vi "XML Script - MathScript Call By Reference Node.vi"(1 "prefix (name)":string, 3 "in":i32=-1, 5 "name":string, 7 "mFilePath":path, 9 "linkIdentity":string, 11 "x":i32=-1, 12 "y":i32=-1, 14 "out":i32=-1) -> (4 "XML Script Command - SubVI":string, 10 "name (wire source)":string)   [LabVIEW 2020]
doc: "linkIdentity: <MFileName>:<FunctionName>\nExample: foo.m:foo"
uses:
  <vilib>/_script/XML Scripting/XML Script Attribute.ctl
  <vilib>/_script/XML Scripting/XML Script Tag.ctl
  <vilib>/_script/XML Scripting/XML Script - PathToXMLString.vi
panel:
  # "position"
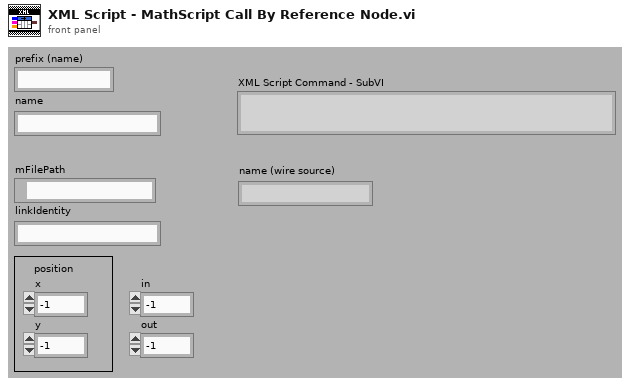
[diagram p1: front panel]
types:
  T1 = typedef "XML Script Attribute.ctl" = enum16{"name", "style", "path", "position", "in", "out", "width", "height", "index", "value", "default", "location", "offset", "typeindex", "size", "source", "destination", "indicator", "type", "controlname", "label", "conpaneidx", "mode", "description", "hasCondTerm", "linkIdentity", "caseselectortype", "concatInputs", "inName", "instantiationpath", "loopCondition", "IndexMode", "formulaInputs", "formulaOutputs", "msnFuncName", "msnIsDynamic", "msnIsODEUserFunction", "ignoreSearchDialog"}
  T2 = typedef "XML Script Tag.ctl" = enum16{"Script", "Function", "SubVI", "GrowableFunction", "Structure", "MultiframeStructure", "Frame", "Tunnel", "ShiftRegister", "Constant", "Control", "Terminal", "Wire", "StaticVIReference", "ControlTerminal", "CompoundArithmetic", "FlatSequence", "FlatSequenceFrame", "MathScriptCallByRef", "BuildArray", "GenericSubVI", "MathScriptNode"}
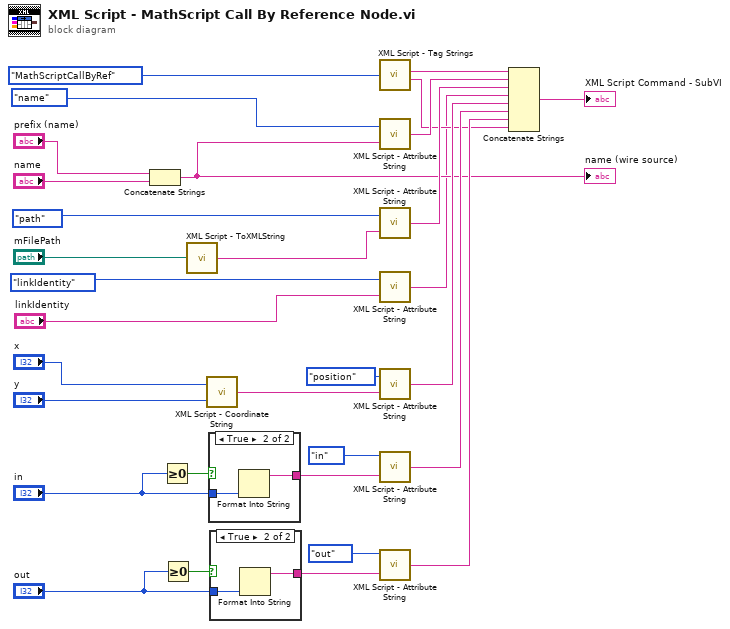
[diagram p0: block diagram]
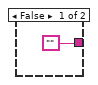
[diagram p2: hidden frame]
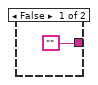
[diagram p3: hidden frame]
diagram:
  n1 = Concatenate Strings("prefix (name)", "name") -> (w7:string)
  "name (wire source)" <- w7
  n2 = Greater Or Equal To 0?(x="in") -> (x >= 0?=w24:bool)
  n3 = Greater Or Equal To 0?(x="out") -> (x >= 0?=w27:bool)
  n4 = call-poly <vilib>:"XML Script - ToXMLString.vi"("Path"="mFilePath") -> ("Valid XML String (out)"=w2:string)
  n5 = call <vilib>:"XML Script - Coordinate String.vi"("y"="y", "x"="x") -> ("(x,y)"=w31:string)
  n6 = case shown="True" w24 {
    tunnel: "in" -> [_ w34]
    tunnel: ["" w33] -> w26
    frame False {
    }
    frame True {
      n7 = Format Into String(w34) -> (resulting string=w33:string)  [unwired: 3 in, 1 out]
    }
  }
  n8 = case shown="True" w27 {
    tunnel: "out" -> [_ w37]
    tunnel: ["" w36] -> w29
    frame False {
    }
    frame True {
      n9 = Format Into String(w37) -> (resulting string=w36:string)  [unwired: 3 in, 1 out]
    }
  }
  n10 = call <vilib>:"XML Script - Tag Strings.vi"("XML Script Tag"=XML_Script_Tag."MathScriptCallByRef") -> ("XML String - Begin Tag"=w14:string, "XML String - End Tag"=w8:string)  [unwired: 2 in]
  n11 = call <vilib>:"XML Script - Attribute String.vi"("Attribute String"=w7, "XML Script Attribute"=XML_Script_Attribute."name") -> ("XML Script - Attribute String"=w13:string)
  n12 = call <vilib>:"XML Script - Attribute String.vi"("Attribute String"=w2, "XML Script Attribute"=XML_Script_Attribute."path") -> ("XML Script - Attribute String"=w12:string)
  n13 = call <vilib>:"XML Script - Attribute String.vi"("Attribute String"="linkIdentity", "XML Script Attribute"=XML_Script_Attribute."linkIdentity") -> ("XML Script - Attribute String"=w3:string)
  n14 = call <vilib>:"XML Script - Attribute String.vi"("Attribute String"=w31, "XML Script Attribute"=XML_Script_Attribute."position") -> ("XML Script - Attribute String"=w11:string)
  n15 = call <vilib>:"XML Script - Attribute String.vi"("Attribute String"=w26, "XML Script Attribute"=XML_Script_Attribute."in") -> ("XML Script - Attribute String"=w10:string)
  n16 = call <vilib>:"XML Script - Attribute String.vi"("Attribute String"=w29, "XML Script Attribute"=XML_Script_Attribute."out") -> ("XML Script - Attribute String"=w9:string)
  n17 = Concatenate Strings(w14, w13, w12, w3, w11, w10, w9, w8) -> (→"XML Script Command - SubVI":string)
